vi "String - (HH_colon_MM) to Minutes.vi"(11 "Hold Time (HH:MM)":string) -> (3 "minutes":dbl)   [LabVIEW 2013]
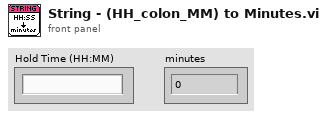
[diagram p1: front panel]
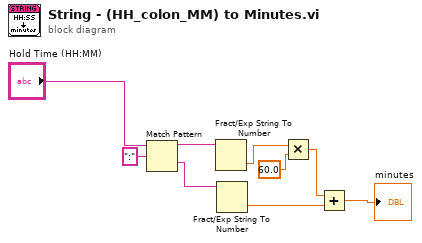
[diagram p0: block diagram]
diagram:
  n1 = Match Pattern(string="Hold Time (HH:MM)", regular expression=":") -> (before substring=w2:string, after substring=w3:string)  [unwired: 1 in, 2 out]
  n2 = Fract/Exp String To Number(string=w2) -> (number=w7:dbl)  [unwired: 3 in, 1 out]
  n3 = Fract/Exp String To Number(string=w3) -> (number=w6:dbl)  [unwired: 3 in, 1 out]
  n4 = Multiply(x=w7, y=60.0) -> (x*y=w5:dbl)
  n5 = Add(x=w5, y=w6) -> (x+y=→"minutes":dbl)
